vi "ABR-Averager.vi"(0 "Runtime":T2, 2 "queue":refnum<queue>, 7 "raw data file":refnum<file>, 9 "Output Scaling":enum16{"Volts", "mV", "uV"}(ring)=enum."uV", 11 "error in (no error)":errorcluster) -> (3 "Rej Thresh out":dbl=15.0, 4 "Runtime thru":T2, 8 "result":T1, 14 "abort":bool, 15 "error out":errorcluster)   [LabVIEW 2020]
uses:
  Typedefs/ABR-Runtime Data.ctl
  epl-vi-lib/Signal Synthesis VIs/4th Generation/Classes/SignalManager/SignalManager.lvclass
  Typedefs/ABR-Queue Data.ctl
  Typedefs/ABR-Parameters.ctl
  Typedefs/ABR-Stimulus.ctl
  Typedefs/ABR-Sequence.ctl
  Typedefs/ABR-Response.ctl
  Threshold Estimation VIs/ABR3-Threshold Estimation Parameters.ctl
  Typedefs/ABR-Averaging Result.ctl
  epl-vi-lib/PXI DAQ VIs/AIDI/Typedefs/AIDI-Action.ctl
  epl-vi-lib/PXI DAQ VIs/AODO/Typedefs/AODO-Action.ctl
  epl-vi-lib/Utility VIs/Conversion VIs/Create Waveform Cluster (2D).vi
panel:
  out "Error":bool
  in  "Reject Override":bool
  in  "Rej Thresh µV":dbl=15.0
  out "Reject":bool
  out "Average":cluster{"offset":dbl, "dx":dbl, "Y":dbl[][]}(graph)
  out "#Aves":i32=120
  out "#Tries":i32=120
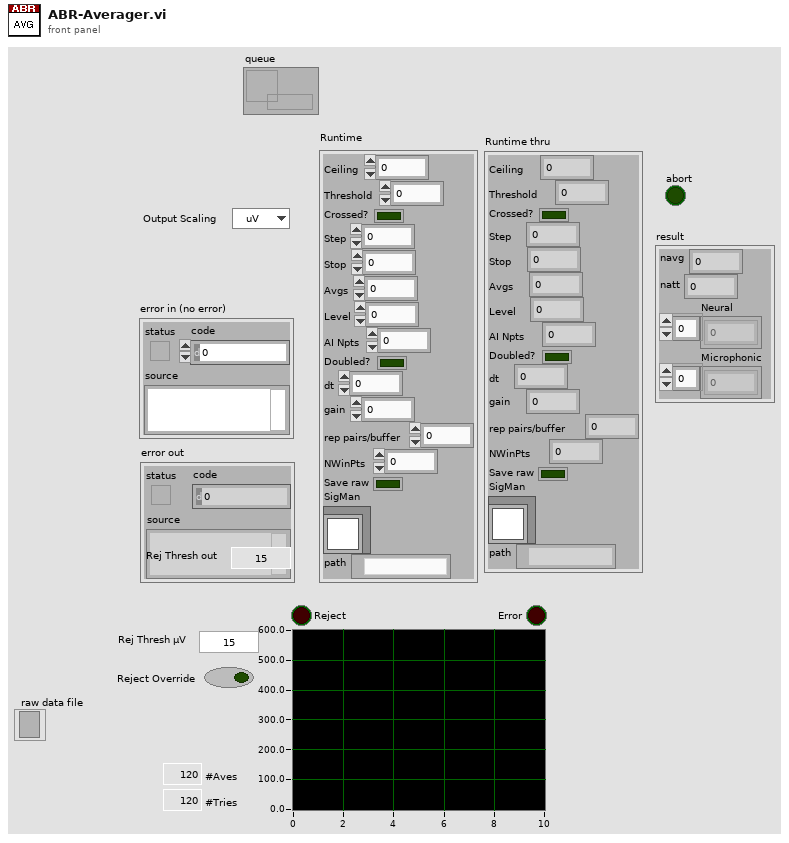
[diagram p1: front panel]
types:
  T1 = typedef "ABR-Averaging Result.ctl" = cluster{"navg":i32, "natt":i32, "Neural":dbl[], "Microphonic":dbl[]}
  T2 = typedef "ABR-Runtime Data.ctl" = cluster{"Ceiling":dbl, "Threshold":dbl, "Crossed?":bool, "Step":dbl, "Stop":i32, "Avgs":i32, "Level":dbl, "AI Npts":i32, "Doubled?":bool, "dt":dbl, "gain":dbl, "rep pairs/buffer":i32, "NWinPts":i32, "Save raw":bool, "SigMan":refnum<class "SignalManager.lvclass">, "path":path}
  T3 = typedef "AODO-Action.ctl" = enum16{"Configure", "Initialize", "Start", "Write", "Clean up", "Init & Start", "Config & Test", "Position", "Set AO Gains", "Zero", "Prime", "Status"}
  T4 = typedef "AIDI-Action.ctl" = enum16{"Configure", "Initialize", "Start", "Read", "Clean up", "Init & Start", "Config & Test", "Position", "Skip"}
  T5 = cluster{i32, i32, "Neural":dbl[], "Microphonic":dbl[]}
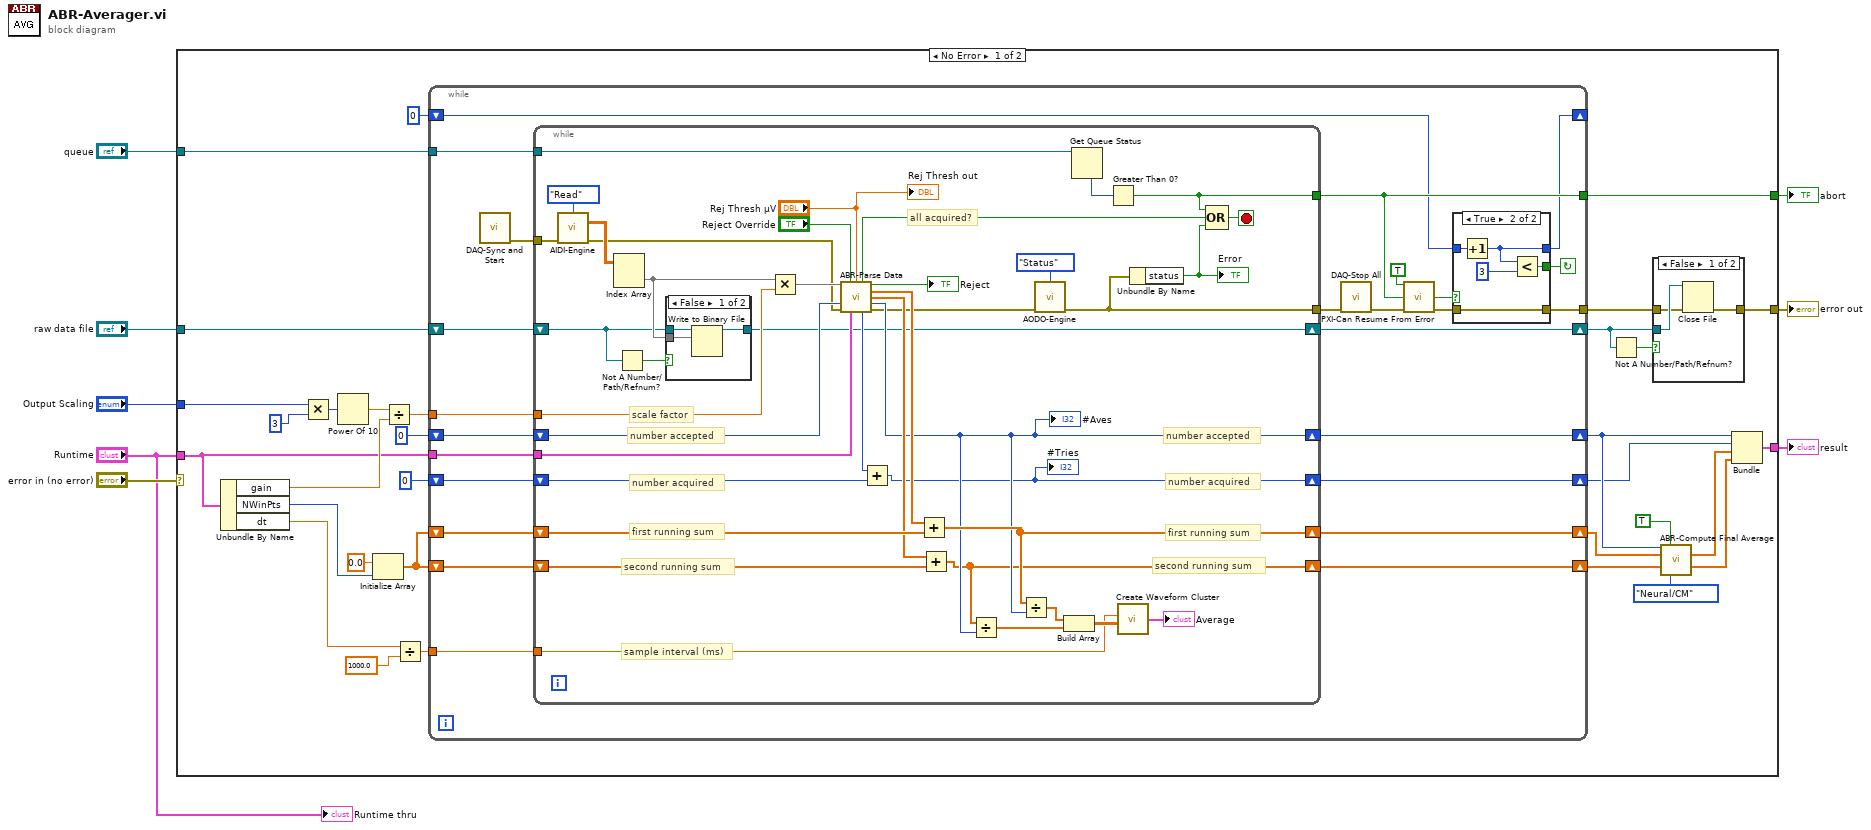
[diagram p0: block diagram]
diagram:
  n1 = case shown="No Error" "error in (no error)" {
    selector: "error in (no error)" -> [_ w120]
    tunnel: "Output Scaling" -> [w36 _]
    tunnel: "Runtime" -> [w26 _]
    tunnel: [w17 w120] -> w7
    tunnel: [w21 _] -> w1
    tunnel: "raw data file" -> [w19 _]
    tunnel: "queue" -> [w14 _]
    tunnel: [w13 _] -> w2
    frame No Error {
      n2 = Unbundle By Name(w26) -> ("gain"=w30:dbl, "NWinPts"=w25:i32, "dt"=w29:dbl)
      n3 = Multiply(x=w36, y=3) -> (x*y=w33:i32)
      n4 = Power Of 10(x=w33) -> (10^x=w34:dbl)
      n5 = Initialize Array(0.0, w25) -> (w28:dbl[])
      n6 = Divide(x=w34, y=w30) -> (x/y=w39:dbl)
      n7 = Divide(x=w29, y=1000.0) -> (x/y=w31:dbl)
      n8 = while {
        tunnel: w39 -> [w65]
        tunnel: w31 -> [w61]
        tunnel: [w41] -> w18
        shift-right: [w62] -> w24
        shift-left: w28 -> [w55]
        shift-right: [w63] -> w37
        shift-left: w28 -> [w54]
        shift-right: [w59] -> w22
        shift-left: 0 -> [w53]
        shift-right: [w60] -> w23
        shift-left: 0 -> [w64]
        tunnel: w26 -> [w52]
        shift-right: [w49] -> w16
        shift-left: w19 -> [w50]
        tunnel: w14 -> [w48]
        tunnel: [w47] -> w13
        shift-right: [w43] -> _
        shift-left: 0 -> [w44]
        stop <- w42 continue-if-true
        n9 = call "DAQ-Sync and Start.vi"() -> ("error out"=w58:errorcluster)  [unwired: 15 in]
        n10 = while {
          shift-right: [w91] -> w63
          shift-left: w54 -> [w109]
          shift-right: [w84] -> w62
          shift-left: w55 -> [w111]
          tunnel: w65 -> [w104]
          shift-right: [w90] -> w60
          shift-left: w64 -> [w96]
          tunnel: w61 -> [w105]
          tunnel: [w102] -> w56
          tunnel: w58 -> [w101]
          shift-right: [w86] -> w59
          shift-left: w53 -> [w99]
          tunnel: w52 -> [w85]
          shift-right: [w81] -> w49
          shift-left: w50 -> [w80]
          tunnel: w48 -> [w76]
          tunnel: [w74] -> w47
          stop <- w106 stop-if-true
          # "scale factor"
          # "all acquired?"
          # "number acquired"
          # "number acquired"
          # "number accepted"
          # "number accepted"
          # "second running sum"
          # "first running sum"
          # "sample interval (ms)"
          # "second running sum"
          # "first running sum"
          n11 = call "AIDI-Engine.vi"("Action"=AIDI-Action."Read", "error in (no error)"=w101) -> ("AI"=w103:dbl[][], "error out"=w77:errorcluster)  [unwired: 8 in, 4 out]
          n12 = Index Array(array=w103) -> (element=w82:dbl[])  [unwired: 2 in]
          n13 = Not A Number/Path/Refnum?(number/path/refnum=w80) -> (NaN/Path/Refnum?=w79:bool)
          n14 = case shown="False" w79 {
            tunnel: w80 -> [w114 w115]
            tunnel: w82 -> [w113 _]
            tunnel: [w112 w115] -> w81
            frame False {
              n15 = Write to Binary File(file (use dialog)=w114, data=w113) -> (refnum out=w112:refnum<file>)  [unwired: 4 in, 2 out]
            }
            frame True {
            }
          }
          n16 = Multiply(x=w82, y=w104) -> (x*y=w83:dbl[])
          n17 = call "ABR-Parse Data.vi"("Data"=w83, "Reject OverRide"="Reject Override", "Rej Thresh µV"="Rej Thresh µV", "Acquired In"=w96, "error in (no error)"=w77, "Runtime"=w85) -> ("Finished?"=w88:bool, "Any rejected?"=→"Reject":bool, "RunSum1"=w94:dbl[], "RunSum2"=w93:dbl[], "Acquired Out"=w90:i32, "Ntries"=w87:i32, "error out"=w89:errorcluster)  [unwired: 3 in]
          "#Aves" <- w90
          n18 = Add(x=w87, y=w99) -> (x+y=w86:i32)
          "#Tries" <- w86
          n19 = Add(x=w94, y=w109) -> (x+y=w91:dbl[])
          n20 = Add(x=w93, y=w111) -> (x+y=w84:dbl[])
          n21 = Divide(x=w84, y=w90) -> (x/y=w110:dbl[])
          n22 = Divide(x=w91, y=w90) -> (x/y=w108:dbl[])
          n23 = call "AODO-Engine.vi"("Action"=AODO-Action."Status", "error in (no error)"=w89) -> ("error out"=w102:errorcluster)  [unwired: 8 in, 5 out]
          n24 = Build Array(w108, w110) -> (w107:dbl[][])
          n25 = Get Queue Status(queue=w76) -> (# elements in queue=w75:i32)  [unwired: 2 in, 7 out]
          n26 = Greater Than 0?(x=w75) -> (x > 0?=w74:bool)
          n27 = call-poly "Create Waveform Cluster.vi"("dx"=w105, "Array"=w107) -> ("waveform cluster"=→"Average":cluster{"offset":dbl, "dx":dbl, "Y":dbl[][]})  [unwired: 3 in]
          n28 = Unbundle By Name(w102) -> ("status"=w100:bool)
          "Error" <- w100
          n29 = Compound Arithmetic op=OR(w74, w88, w100) -> (w106:bool)
          "Rej Thresh out" <- "Rej Thresh µV"
        }
        n30 = call "DAQ-Stop All.vi"("error in (no error)"=w56) -> ("error out"=w57:errorcluster)  [unwired: 14 in]
        n31 = call "PXI-Can Resume From Error.vi"("Ignore local?"=TRUE, "Abort"=w47, "error in (no error)"=w57) -> ("Resume?"=w45:bool, "error out"=w46:errorcluster)  [unwired: 10 in, 1 out]
        n32 = case shown="True" w45 {
          tunnel: w46 -> [w66 w68]
          tunnel: w44 -> [w67 w72]
          tunnel: [w67 w71] -> w43
          tunnel: [_ w69] -> w42
          tunnel: [w66 w68] -> w41
          frame False {
          }
          frame True {
            n33 = Increment(x=w72) -> (x+1=w71:i32)
            n34 = Less?(x=w71, y=3) -> (x < y?=w69:bool)
          }
        }
      }
      n35 = Not A Number/Path/Refnum?(number/path/refnum=w16) -> (NaN/Path/Refnum?=w15:bool)
      n36 = case shown="False" w15 {
        tunnel: w16 -> [w118 _]
        tunnel: w18 -> [w117 w119]
        tunnel: [w116 w119] -> w17
        frame False {
          n37 = Close File(refnum=w118, error in=w117) -> (error out=w116:errorcluster)  [unwired: 1 out]
        }
        frame True {
        }
      }
      n38 = call "ABR-Compute Final Average.vi"("#Avgs"=w23, "Remove DC Offset"=TRUE, "Running Sum 1"=w37, "Running Sum 2"=w24, "Avg Mode"=enum16{"Neural/CM", "ANOW"}."Neural/CM") -> ("Neural"=w12:dbl[], "Microphonic"=w11:dbl[])  [unwired: 9 in]
      n39 = Bundle(w23, w22, "Neural"=w12, "Microphonic"=w11) -> (w21:T5)  [unwired: 1 in]
    }
    frame Error {
    }
  }
  "error out" <- w7
  "abort" <- w2
  "result" <- w1
  "Runtime thru" <- "Runtime"
